vi "SHTStatusJson.vi"(8 "error in (no error)":errorcluster, 11 "JSON string":string) -> (0 "error out":errorcluster, 3 "value":cluster{"Capteur":string, "status":bool}[](array[cluster]))   [LabVIEW 2018]
panel:
  in  "Array":cluster{"Capteur":string, "Status":bool}[](array[cluster])
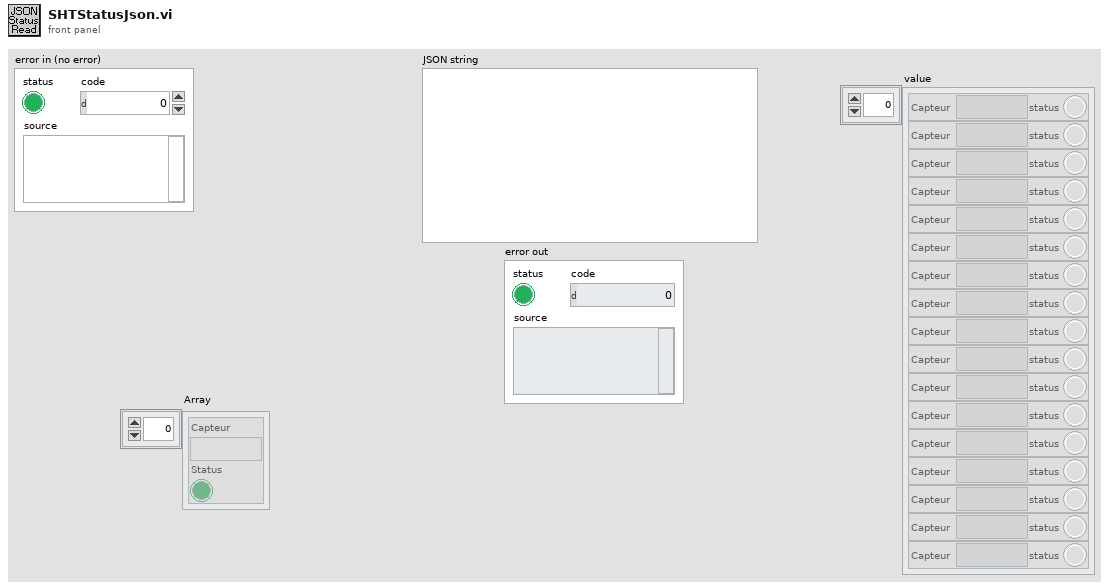
[diagram p1: front panel]
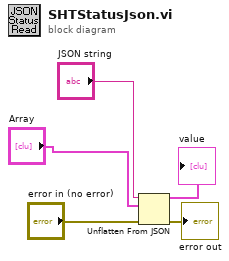
[diagram p0: block diagram]
diagram:
  n1 = Unflatten From JSON(JSON string="JSON string", type and defaults="Array", error in (no error)="error in (no error)") -> (value=→"value":cluster{"Capteur":string, "Status":bool}[], error out=→"error out":errorcluster)  [unwired: 4 in]
